vi "ASIC_CONFIGURAR SALIDAS BUF ENA.vi"(7 "Espera acceso USB":u32=10, 8 "error in":errorcluster, 10 "BUF ENA":bool, 11 "ftHandle_in":u32) -> (0 "error out":errorcluster, 3 "ftHandle_out":u32)   [LabVIEW 2019]
panel:
  out "test":u16 format="%04x"
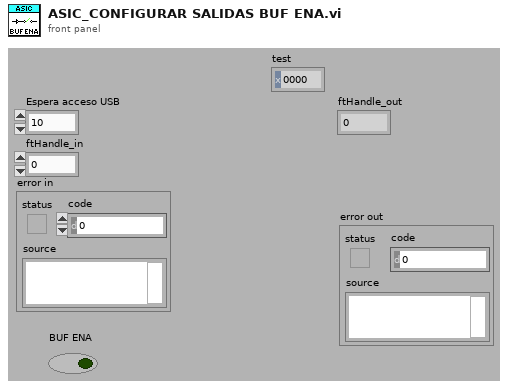
[diagram p1: front panel]
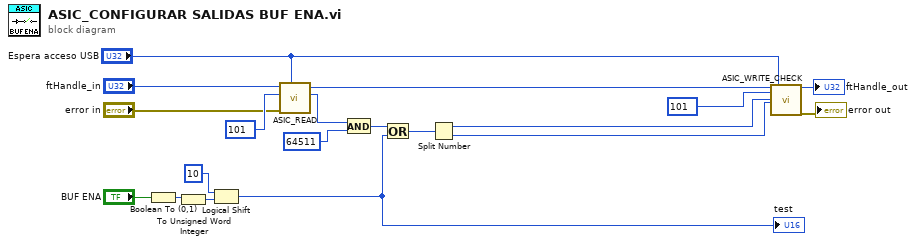
[diagram p0: block diagram]
diagram:
  n1 = Boolean To (0,1)(Boolean="BUF ENA") -> (0, 1=w4:i16)
  n2 = To Unsigned Word Integer(number=w4) -> (unsigned 16bit integer=w3:u16)
  n3 = Logical Shift(y=u16 10 ("x"), x=w3) -> (x << y=w1:u16)
  "test" <- w1
  n4 = call "ASIC_READ.vi"("Espera acceso USB"="Espera acceso USB", "error in"="error in", "Direccion Registro Asic"=u8 101, "ftHandle_in"="ftHandle_in") -> ("Valor Asic"=w9:u16, "ftHandle_out"=w12:u32)  [unwired: 5 in, 1 out]
  n5 = And(x=w9, y=u16 64511) -> (x .and. y?=w7:u16)
  n6 = Or(x=w7, y=w1) -> (x .or. y?=w6:u16)
  n7 = Split Number(x=w6) -> (hi(x)=w11:u8, lo(x)=w10:u8)
  n8 = call "ASIC_WRITE_CHECK.vi"("ftHandle_in"=w12, "Direccion Registro Asic"=u8 101, "Byte Alto"=w11, "Byte Bajo"=w10, "Espera acceso USB 2"="Espera acceso USB") -> ("ftHandle_out"=→"ftHandle_out":u32, "error out"=→"error out":errorcluster)  [unwired: 12 in, 1 out]
